vi "cdaq_anal_adc_capture.vi"(8 "error in":errorcluster, 10 "N":i32, 11 "cdaq session in":T1={"mclk [Hz]"=12800000.0, "DAC device"="", "ADC device"="", "DAC task"="", "ADC task"="", "adc idn"="", "dac idn"="", "fs [Hz]"=50000.0, "queue adc cmd"=refnum, "queue adc data"=refnum, "adc proc ref"=refnum}) -> (0 "error out":errorcluster, 1 "timestamp [s]":dbl, 2 "wave":dbl[](array[numeric]), 3 "cdaq session out":T1={"mclk [Hz]"=12800000.0, "DAC device"="", "ADC device"="", "DAC task"="", "ADC task"="", "adc idn"="", "dac idn"="", "fs [Hz]"=50000.0, "queue adc cmd"=refnum, "queue adc data"=refnum, "adc proc ref"=refnum})   [LabVIEW 2013]
uses:
  cdaq_anal_session.ctl
  cdaq_anal_adc_command.ctl
  cdaq_anal_adc_data.ctl
  <vilib>/Utility/error.llb/Error Cluster From Error Code.vi
  <vilib>/ErrorRing/Error Ring.xnode
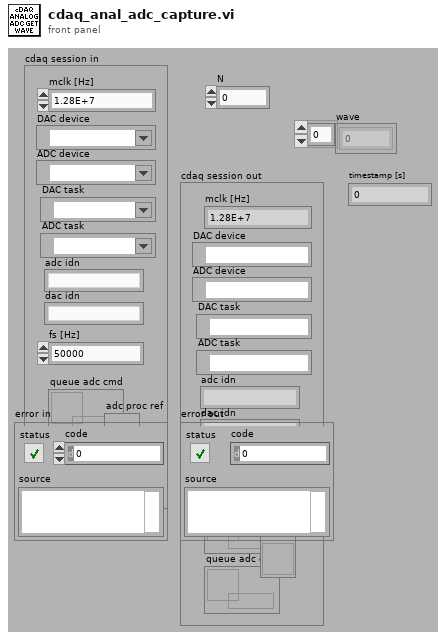
[diagram p1: front panel]
types:
  T1 = typedef "cdaq_anal_session.ctl" = cluster{"mclk [Hz]":dbl, "DAC device":tag, "ADC device":tag, "DAC task":refnum<k21>, "ADC task":refnum<k21>, "adc idn":string, "dac idn":string, "fs [Hz]":dbl, "queue adc cmd":refnum<queue>, "queue adc data":refnum<queue>, "adc proc ref":refnum<vi>}
  T2 = typedef "cdaq_anal_adc_command.ctl" = cluster{"sample to get":i32, "stop":bool}
  T3 = typedef "cdaq_anal_adc_data.ctl" = cluster{"wave":dbl[], "timestamp [s]":dbl}
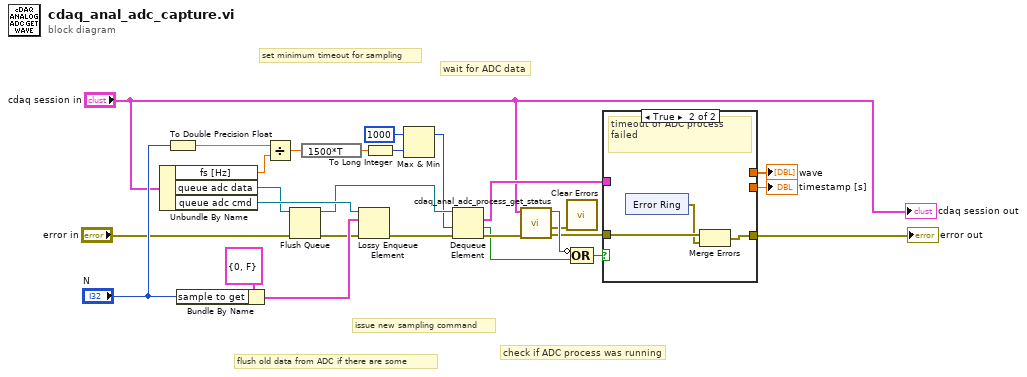
[diagram p0: block diagram]
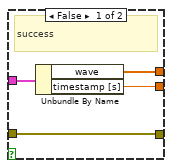
[diagram p2: hidden frame]
diagram:
  # "check if ADC process was running"
  # "set minimum timeout for sampling"
  # "wait for ADC data"
  # "issue new sampling command"
  # "flush old data from ADC if there are some"
  n1 = Unbundle By Name("cdaq session in") -> ("fs [Hz]"=w22:dbl, "queue adc data"=w18:refnum<queue>, "queue adc cmd"=w26:refnum<queue>)
  n2 = To Double Precision Float(number="N") -> (double precision float=w23:dbl)
  n3 = Bundle By Name(cluster=T2 {"sample to get"=0, "stop"=FALSE} ("adc cmd"), "sample to get"="N") -> (w25:T2)
  n4 = Divide(x=w23, y=w22) -> (x/y=w21:dbl)
  n5 = Flush Queue(queue=w18, error in (no error)="error in") -> (queue out=w16:refnum<queue>, error out=w20:errorcluster)  [unwired: 1 out]
  n6 = expression code="1500*T"(w21) -> (w15:dbl)
  n7 = Lossy Enqueue Element(queue=w26, element=w25, error in (no error)=w20) -> (error out=w17:errorcluster)  [unwired: 3 out]
  n8 = To Long Integer(number=w15) -> (32bit integer=w14:i32)
  n9 = Max & Min(x=1000, y=w14) -> (max(x,y)=w12:i32)  [unwired: 1 out]
  n10 = Dequeue Element(queue=w16, timeout in ms (-1)=w12, error in (no error)=w17) -> (element=w4:T3, timed out?=w10:bool, error out=w11:errorcluster)  [unwired: 1 out]
  n11 = call "cdaq_anal_adc_process_get_status.vi"("error in"=w11, "cdaq session"="cdaq session in") -> ("error out"=w7:errorcluster, "sweep error out"=w6:errorcluster, "is running"=w9:bool)  [unwired: 7 in]
  n12 = call <vilib>:"Clear Errors.vi"("error in (no error)"=w6) -> ()  [unwired: 6 in, 1 out]
  n13 = Compound Arithmetic op=OR(invert w9, w10) -> (w8:bool)
  n14 = case shown="True" w8 {
    tunnel: w7 -> [w31 w34]
    tunnel: [w31 w32] -> w5
    tunnel: w4 -> [w30 _]
    tunnel: [w29 _] -> w3
    tunnel: [w28 _] -> w1
    frame False {
      # "success"
      n15 = Unbundle By Name(w30) -> ("wave"=w29:dbl[], "timestamp [s]"=w28:dbl)
    }
    frame True {
      # "timeout or ADC process failed"
      n16 = xnode "Error Ring"() -> ("error out"=w33:errorcluster)
      n17 = Merge Errors(w34, w33) -> (w32:errorcluster)
    }
  }
  "error out" <- w5
  "wave" <- w3
  "timestamp [s]" <- w1
  "cdaq session out" <- "cdaq session in"
